vi "string methods.vi"() -> ()   [LabVIEW 2024]
panel:
  out "result string 2":string
  in  "replace string (\"\")":string
  in  "search string":string
  out "replaced substring":string
  out "result string":string
  in  "length (len. of substring)":i32
  in  "offset (0) 2":i32
  in  "substring (\"\")":string
  out "substring":string
  in  "length (rest)":i32
  in  "offset (0)":i32
  out "length":i32
  in  "String":string
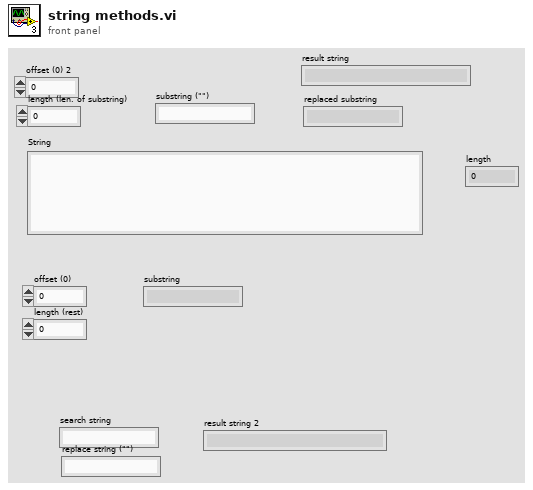
[diagram p1: front panel]
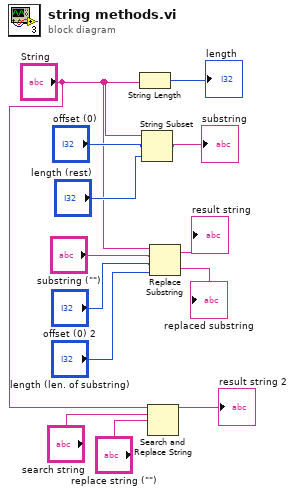
[diagram p0: block diagram]
diagram:
  n1 = String Length(string="String") -> (length=→"length":i32)
  n2 = String Subset(string="String", offset (0)="offset (0)", length (rest)="length (rest)") -> (substring=→"substring":string)
  n3 = Search and Replace String(input string="String", search string="search string", replace string="replace string (\"\")") -> (result string=→"result string 2":string)  [unwired: 5 in, 3 out]
  n4 = Replace Substring(2:"length (len. of substring)", 3:"offset (0) 2", 4:"substring (\"\")", 5:"String") -> (0:→"replaced substring":string, 1:→"result string":string)
